vi "FTW-dotNET-SQL-ExecuteScript.vi"(0 "DB Connection":refnum<k24>, 5 "SQL Script":string, 11 "error in":errorcluster) -> (4 "DB Connection out":refnum<k24>, 6 "Elapsed Time":dbl format="%.4psec", 15 "error out":errorcluster)   [LabVIEW 2015]
uses:
  System.Data
panel:
  # "Inputs"
  # "Outputs"
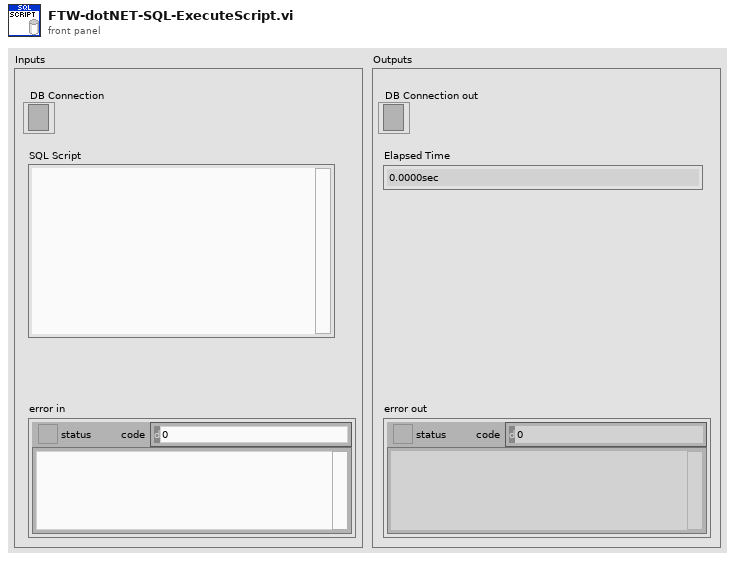
[diagram p1: front panel]
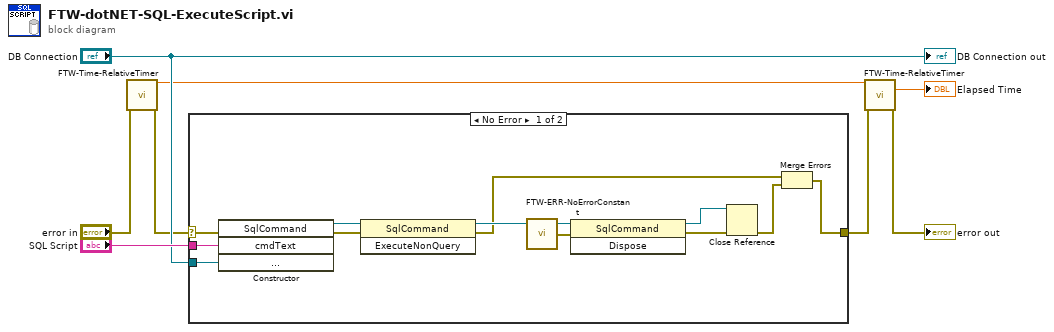
[diagram p0: block diagram]
diagram:
  n1 = call "FTW-Time-RelativeTimer.vi"("error in"="error in") -> ("Current Timer Value"=w4:dbl, "error out"=w5:errorcluster)  [unwired: 12 in, 1 out]
  n2 = case shown="No Error" w5 {
    selector: w5 -> [w10 w21]
    tunnel: "SQL Script" -> [w11 _]
    tunnel: [w12 w21] -> w1
    tunnel: "DB Connection" -> [w18 _]
    frame No Error {
      n3 = constructor class="SqlCommand"(error in=w10, "cmdText"=w11, "connection"=w18) -> (reference out=w20:refnum<k24>, error out=w19:errorcluster)  [unwired: 2 in, 3 out]
      n4 = invoke on="Invoke Node" class="SqlCommand" method="ExecuteNonQuery"(reference=w20, error in=w19) -> (reference out=w14:refnum<k24>, error out=w9:errorcluster)  [unwired: 1 in, 1 out]
      n5 = call "FTW-ERR-NoErrorConstant.vi"() -> ("no error"=w15:errorcluster)
      n6 = invoke class="SqlCommand" method="Dispose"(reference=w14, error in=w15) -> (reference out=w16:refnum<k24>, error out=w17:errorcluster)  [unwired: 1 in, 1 out]
      n7 = Close Reference(reference=w16, error in (no error)=w17) -> (error out=w13:errorcluster)
      n8 = Merge Errors(w9, w13) -> (w12:errorcluster)
    }
    frame Error {
    }
  }
  n9 = call "FTW-Time-RelativeTimer.vi"("Previous Timer Value"=w4, "error in"=w1) -> ("Elapsed Time"=→"Elapsed Time":dbl, "error out"=→"error out":errorcluster)  [unwired: 11 in, 1 out]
  "DB Connection out" <- "DB Connection"
